vi "Read Lock-in.vi"(8 "error in (no error)":errorcluster, 11 "Lock-in Command Msg in":refnum<class "Lock-in Command Msg.lvclass">) -> (0 "error out":errorcluster, 2 "Lock-in":bool, 3 "Lock-in Command Msg out":refnum<class "Lock-in Command Msg.lvclass">)   [LabVIEW 2021, in "Lock-in Command Msg.lvclass"]
uses:
  Lock-in Command Msg.lvclass
  Lock-in Command Msg.lvclass/Lock-in Command Msg.ctl
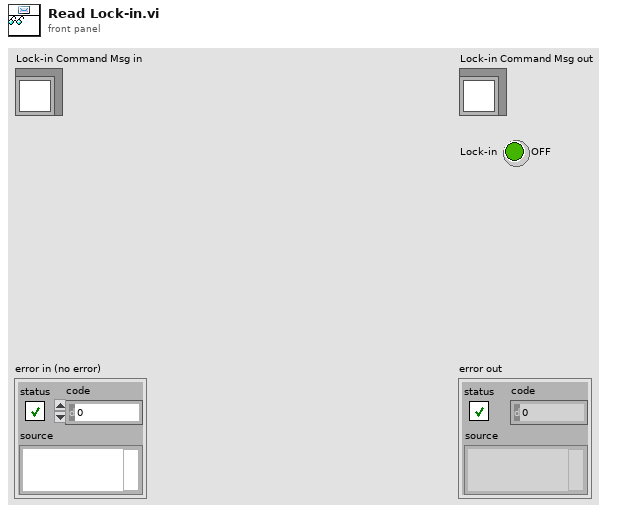
[diagram p1: front panel]
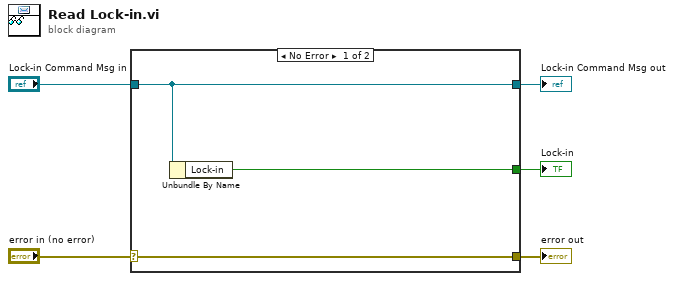
[diagram p0: block diagram]
diagram:
  n1 = case shown="No Error" "error in (no error)" {
    selector: "error in (no error)" -> [w8 w9]
    tunnel: [w8 w9] -> w4
    tunnel: [w7 w10] -> w2
    tunnel: "Lock-in Command Msg in" -> [w7 w10]
    tunnel: [w6 _] -> w1
    frame No Error {
      n2 = Unbundle By Name(w7) -> ("Lock-in"=w6:bool)
    }
    frame Error {
    }
  }
  "error out" <- w4
  "Lock-in Command Msg out" <- w2
  "Lock-in" <- w1
